vi "AnalogIntegrator_NI5771.vi"() -> ()   [LabVIEW 2012]
uses:
  <vilib>/Platform/TimedLoop/XDataNode/timing_clust.ctl
  <vilib>/Platform/TimedLoop/XDataNode/nitl_modes.ctl
  <vilib>/Platform/TimedLoop/XDataNode/wakeup.ctl
  <vilib>/rvi/FIFO/Fifo_Resource/nirvififoEmulationSetSize.vi
  <vilib>/rvi/DataTransferAndStorage/Container/Common/niFpgaContainerGetUniqueNameForEmu.vi
  <vilib>/rvi/eio/common/nirviEmuTemplateMethod_errors.vi
  <vilib>/rvi/Emulation/niFpgaSctlEmulationRegisterWithScheduler.vi
  <vilib>/rvi/errors/niFpgaSetErrorForExecOnDevCompSimple.vi
  <vilib>/rvi/eio/common/nirviEmuReportErrorAndStop.vi
  <vilib>/rvi/Emulation/niFpgaSctlEmulationFifoFullMgr.vi
  <vilib>/rvi/Emulation/niFpgaSctlEmulationResourceMgr.vi
  <vilib>/rvi/Emulation/niFpgaSctlEmulationScheduler.vi
  <vilib>/rvi/interface/RandomDataEmulation/nirviRandomDataFPGAFIFO.vi
  <vilib>/rvi/interface/RandomDataEmulation/niFpgaRandomDataHandleErrors.vi
  <vilib>/rvi/Emulation/niFpgaSctlEmulationGlobalWrite.vi
  <vilib>/Platform/TimedLoop/XDataNode/XDataNode.xnode
  <vilib>/rvi/DataTransferAndStorage/Container/XNode/niFpgaContainer.xnode
  <vilib>/rvi/FIFO/Fifo_Resource/nirvififoEmulationClear.vi
  <vilib>/eio/EIONode/EIONode.xnode
  <vilib>/rvi/FIFO/Fifo_Resource/nirvififoEmulationWrite.vi
  <vilib>/rvi/FIFO/Fifo_Resource/nirvififoEmulationRead.vi
  <vilib>/rvi/interface/RandomDataEmulation/nirviRandomDataFpgaReadWriteTemplate.vi
  <vilib>/Platform/TimedLoop/XDataNode/XDNodeRunTimeDep.lvlib
panel:
  in  "Baselinex8 Ch2":u8
  in  "Baselinex8 Ch1":u8
  in  "Clear Interloop FIFO":bool
  out "InterloopFIFO Timeout":bool
  out "ToHostCh2FIFO Overflow":bool
  out "ToHostCh1FIFO Overflow":bool
  out "Pixel counter":u32
  in  "Wait for trigger":bool
  in  "Acquire":bool
  in  "Acquire continuously":bool=TRUE
  in  "Requested pixels":u32=100000
  out "InterloopFIFO Overflow":bool
  out "Acquiring":bool
  out "IO Module\\AI Over Range":bool
  in  "Samples per pixel":u32=10000 caption="Samples per pixel Acq"
  in  "Samples per line":u32=10000 caption="Samples per pixel Acq"
  in  "User Command Commit":bool
  in  "User Command":u8
  out "User Command Idle":bool
  out "User Command Status":u8
  in  "User Data 0":u16
  in  "User Data 1":u8
  out "PLL Locked":bool
  out "User Error":bool
  out "Configured?":bool
  # "5771 IO module configuration"
  # "Analog integrator"
  # "Acquisition control"
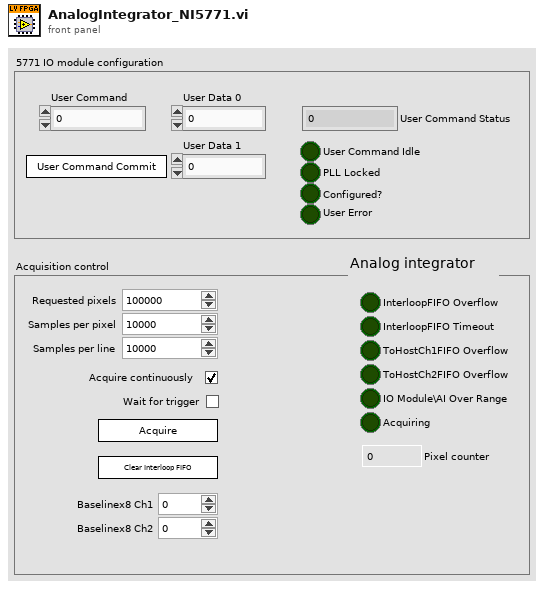
[diagram p1: front panel]
types:
  T1 = typedef "XDNodeRunTimeDep.lvlib/timing_clust.ctl" = cluster{"Expected End [f-1]":u64, "Actual End [f-1]":u64, "Finished Late? [f-1]":bool, "Expected End [i-1]":u64, "Actual End [i-1]":u64, "Finished Late? [i-1]":bool, "Expected Start [i]":u64, "Actual Start [i]":u64, "Expected Start [f]":u64, "Actual Start [f]":u64, "Source Name":string, "Structure Name":string, "Period":i64, "Deadline":i64, "Offset":i64, "Start":i64, "Priority":i32, "Timeout":i32, "Mode":T2, "Wakeup Reason":T3, "Error":errorcluster, "Source Type":string, "Secondary Source Type":string, "Global End Time":u64, "Global Start Time":u64, "Frame Duration":u64, "Iteration Duration":u64, "Assigned CPU":i32, "I/O Scan Engine Mode":u32}
  T2 = typedef "XDNodeRunTimeDep.lvlib/nitl_modes.ctl" = enum32{"No Change", "Process missed periods, maintain original phase", "Discard missed periods, maintain original phase", "Process missed periods, ignore original phase", "Discard missed periods, ignore original phase"}
  T3 = typedef "XDNodeRunTimeDep.lvlib/wakeup.ctl" = enum32{"Normal", "Aborted", "Asynchronous wakeup", "Timing source error", "Timed loop error", "Timeout"}
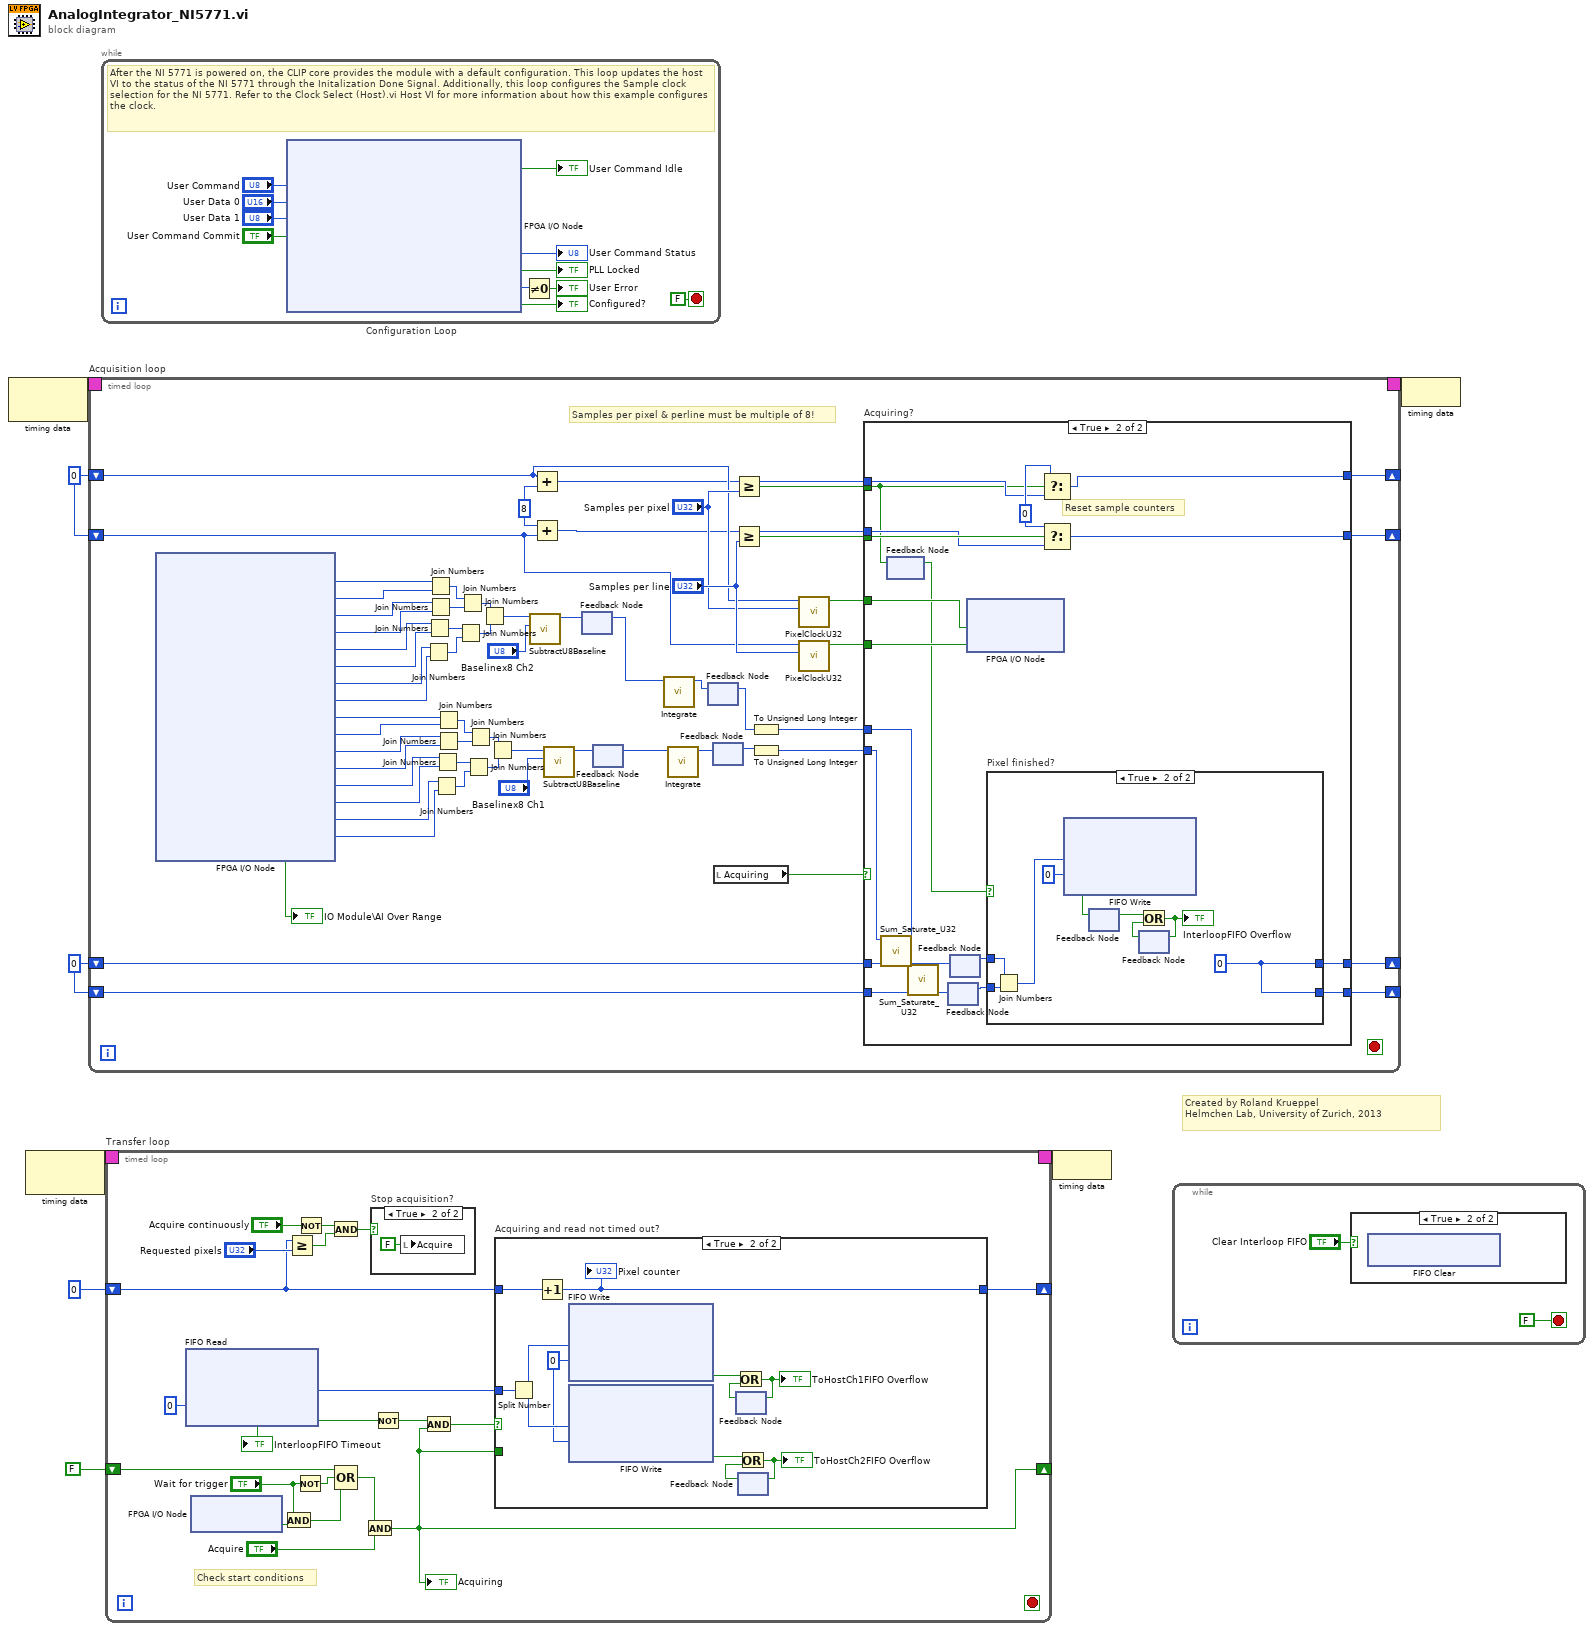
[diagram p0: block diagram]
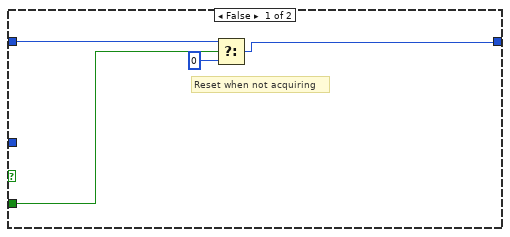
[diagram p4: hidden frame]
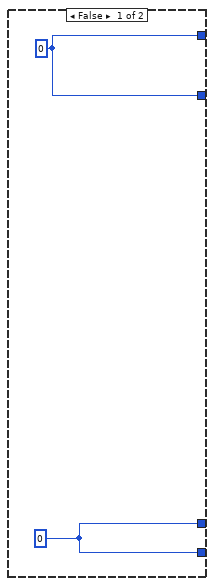
[diagram p5: hidden frame]
diagram:
  w5 = u32 0
  w6 = u32 0 ("t")
  # "Created by Roland Krueppel\nHelmchen Lab, University of Zurich, 2013"
  n1 = node-c288() -> (w8:T1)  [unwired: 1 in]
  n2 = node-c288() -> (w4:T1)  [unwired: 1 in]
  n3 = timed-loop "Acquisition loop" {
    timing: w8 -> [_]
    timing-out: [_] -> w7
    shift-right: [w68] -> _
    shift-left: w6 -> [w57]
    shift-right: [w69] -> _
    shift-left: w6 -> [w56]
    shift-right: [w64] -> _
    shift-left: w5 -> [w66]
    shift-right: [w63] -> _
    shift-left: w5 -> [w65]
    stop <- _ stop-if-true
    w60 = u32 8 ("y")
    # "Samples per pixel & perline must be multiple of 8!"
    n4 = xnode "FPGA I/O Node"() -> ("IO Module\\AI 1 Data N-7"=w42:u8, "IO Module\\AI 1 Data N-6"=w41:u8, "IO Module\\AI 1 Data N-5"=w40:u8, "IO Module\\AI 1 Data N-4"=w39:u8, "IO Module\\AI 1 Data N-3"=w38:u8, "IO Module\\AI 1 Data N-2"=w37:u8, "IO Module\\AI 1 Data N-1"=w36:u8, "IO Module\\AI 1 Data N"=w35:u8, "IO Module\\AI 0 Data N-7"=w28:u8, "IO Module\\AI 0 Data N-6"=w27:u8, "IO Module\\AI 0 Data N-5"=w26:u8, "IO Module\\AI 0 Data N-4"=w25:u8, "IO Module\\AI 0 Data N-3"=w24:u8, "IO Module\\AI 0 Data N-2"=w23:u8, "IO Module\\AI 0 Data N-1"=w22:u8, "IO Module\\AI 0 Data N"=w21:u8, "IO Module\\AI Over Range"=→"IO Module\\AI Over Range":bool)  [unwired: 17 in, 17 out]
    n5 = Join Numbers(hi=w36, lo=w35) -> ((hi.lo)=w46:u16)
    n6 = Join Numbers(hi=w38, lo=w37) -> ((hi.lo)=w45:u16)
    n7 = Join Numbers(hi=w42, lo=w41) -> ((hi.lo)=w43:u16)
    n8 = Join Numbers(hi=w40, lo=w39) -> ((hi.lo)=w44:u16)
    n9 = Join Numbers(hi=w22, lo=w21) -> ((hi.lo)=w32:u16)
    n10 = Join Numbers(hi=w24, lo=w23) -> ((hi.lo)=w31:u16)
    n11 = Join Numbers(hi=w28, lo=w27) -> ((hi.lo)=w29:u16)
    n12 = Join Numbers(hi=w26, lo=w25) -> ((hi.lo)=w30:u16)
    n13 = Join Numbers(hi=w45, lo=w46) -> ((hi.lo)=w48:u32)
    n14 = Join Numbers(hi=w43, lo=w44) -> ((hi.lo)=w47:u32)
    n15 = Join Numbers(hi=w31, lo=w32) -> ((hi.lo)=w34:u32)
    n16 = Join Numbers(hi=w29, lo=w30) -> ((hi.lo)=w33:u32)
    n17 = Join Numbers(hi=w47, lo=w48) -> ((hi.lo)=w19:u64)
    n18 = Join Numbers(hi=w33, lo=w34) -> ((hi.lo)=w18:u64)
    n19 = call "SubtractU8Baseline.vi"("Baseline U8"="Baselinex8 Ch2", "New samples in"=w19) -> ("New samples out"=w13:u64)  [unwired: 9 in]
    n20 = Add(x=w56, y=w60) -> (x+y=w53:u32)
    n21 = Add(x=w60, y=w57) -> (x+y=w51:u32)
    n22 = call "SubtractU8Baseline.vi"("Baseline U8"="Baselinex8 Ch1", "New samples in"=w18) -> ("New samples out"=w16:u64)  [unwired: 9 in]
    n23 = feedback-in #1(w13) -> ()
    n24 = feedback #1() -> (w14:u64)  [unwired: 1 in]
    n25 = feedback #2() -> (w15:u64)  [unwired: 1 in]
    n26 = feedback-in #2(w16) -> ()
    n27 = call "Integrate.vi"("New samples in"=w14) -> ("Sum out"=w12:u16)  [unwired: 9 in, 1 out]
    n28 = call "Integrate.vi"("New samples in"=w15) -> ("Sum out"=w10:u16)  [unwired: 9 in, 1 out]
    n29 = feedback #3() -> (w11:u16)  [unwired: 1 in]
    n30 = feedback-in #3(w12) -> ()
    n31 = feedback #4() -> (w9:u16)  [unwired: 1 in]
    n32 = feedback-in #4(w10) -> ()
    n33 = local read "Acquiring"() -> (w67:bool)
    n34 = Greater Or Equal?(x=w53, y="Samples per pixel") -> (x >= y?=w52:bool)
    n35 = Greater Or Equal?(x=w51, y="Samples per line") -> (x >= y?=w50:bool)
    n36 = To Unsigned Long Integer(number=w11) -> (unsigned 32bit integer=w55:u32)
    n37 = To Unsigned Long Integer(number=w9) -> (unsigned 32bit integer=w54:u32)
    n38 = call "PixelClockU32.vi"("Samples per pixel"="Samples per pixel", "Sample counter"=w56) -> ("Pixel clock"=w59:bool)  [unwired: 9 in]
    n39 = call "PixelClockU32.vi"("Samples per pixel"="Samples per line", "Sample counter"=w57) -> ("Pixel clock"=w58:bool)  [unwired: 9 in]
    n40 = case "Acquiring?" shown="True" w67 {
      tunnel: [w71 w90] -> w69
      tunnel: [w71 w89] -> w68
      tunnel: w54 -> [_ w76]
      tunnel: w66 -> [_ w79]
      tunnel: w65 -> [_ w75]
      tunnel: w55 -> [_ w74]
      tunnel: [w70 w88] -> w64
      tunnel: [w70 w87] -> w63
      tunnel: w52 -> [_ w81]
      tunnel: w50 -> [_ w86]
      tunnel: w53 -> [_ w85]
      tunnel: w51 -> [_ w84]
      tunnel: w59 -> [_ w83]
      tunnel: w58 -> [_ w82]
      frame False {
        w70 = u32 0
        w71 = u16 0 ("t")
      }
      frame True {
        w91 = u32 0 ("t")
        # "Reset sample counters"
        n41 = call "Sum_Saturate_U32.vi"("Sum In"=w79, "New Value"=w76) -> ("Sum Out"=w78:u32)  [unwired: 9 in]
        n42 = feedback #5() -> (w80:bool)  [unwired: 1 in]
        n43 = feedback-in #5(w81) -> ()
        n44 = call "Sum_Saturate_U32.vi"("Sum In"=w75, "New Value"=w74) -> ("Sum Out"=w73:u32)  [unwired: 9 in]
        n45 = feedback #6() -> (w72:u32)  [unwired: 1 in]
        n46 = feedback-in #6(w73) -> ()
        n47 = feedback #7() -> (w77:u32)  [unwired: 1 in]
        n48 = feedback-in #7(w78) -> ()
        n49 = xnode "FPGA I/O Node"("PixelClock"=w83, "LineClock"=w82) -> ()  [unwired: 2 in, 2 out]
        n50 = case "Pixel finished?" shown="True" w80 {
          tunnel: w72 -> [w92 w102]
          tunnel: w77 -> [w93 w101]
          tunnel: [w93 w96] -> w88
          tunnel: [w92 w96] -> w87
          frame False {
          }
          frame True {
            w96 = u32 0
            n51 = Join Numbers(hi=w101, lo=w102) -> ((hi.lo)=w100:u64)
            n52 = xnode ("FIFO Write")("Element"=w100, "Timeout"=0) -> ("Timed Out?"=w94:bool)  [unwired: 1 in, 1 out]
            n53 = feedback-in #8(w94) -> ()
            n54 = feedback #8() -> (w95:bool)  [unwired: 1 in]
            n55 = feedback #9() -> (w97:bool)  [unwired: 1 in]
            n56 = Or(x=w95, y=w97) -> (x .or. y?=w98:bool)
            "InterloopFIFO Overflow" <- w98
            n57 = feedback-in #9(w98) -> ()
          }
        }
        n58 = Select(t=w91, s=w81, f=w85) -> (s? t:f=w90:u32)
        n59 = Select(t=w91, s=w86, f=w84) -> (s? t:f=w89:u32)
      }
    }
  }
  n60 = while "Configuration Loop" {
    stop <- FALSE stop-if-true
    # "After the NI 5771 is powered on, the CLIP core provides the module with a default configuration. This loop updates the host VI to the status of the NI 5771 through the Initalization Done Signal. Additionally, this loop configures the Sample clock selection for the NI 5771. Refer to the Clock Select (Host).vi Host VI for more information about how this example configures the clock."
    n61 = xnode "FPGA I/O Node"("IO Module\\User Command"="User Command", "IO Module\\User Data 0"="User Data 0", "IO Module\\User Data 1"="User Data 1", "IO Module\\User Command Commit"="User Command Commit") -> ("IO Module\\User Command Idle"=→"User Command Idle":bool, "IO Module\\User Command Status"=→"User Command Status":u8, "IO Module\\PLL Locked"=→"PLL Locked":bool, "IO Module\\User Error"=w108:u8, "IO Module\\Initialization Done"=→"Configured?":bool)  [unwired: 9 in, 9 out]
    n62 = Not Equal To 0?(x=w108) -> (x != 0?=→"User Error":bool)
  }
  n63 = timed-loop "Transfer loop" {
    timing: w4 -> [_]
    timing-out: [_] -> w3
    shift-right: [w118] -> _
    shift-left: u32 0 -> [w119]
    shift-right: [w117] -> _
    shift-left: FALSE -> [w125]
    stop <- _ stop-if-true
    # "Check start conditions"
    n64 = xnode ("FIFO Read")("Timeout"=0) -> ("Element"=w120:u64, "Timed Out?"=w124:bool)  [unwired: 1 in, 1 out]
    "InterloopFIFO Timeout" <- w124
    n65 = xnode "FPGA I/O Node"() -> ("TriggerIn"=w130:bool)  [unwired: 1 in, 1 out]
    n66 = And(x="Wait for trigger", y=w130) -> (x .and. y?=w127:bool)
    n67 = Greater Or Equal?(x=w119, y="Requested pixels") -> (x >= y?=w132:bool)
    n68 = Not(x="Wait for trigger") -> (.not. x?=w128:bool)
    n69 = Not(x="Acquire continuously") -> (.not. x?=w133:bool)
    n70 = And(x=w133, y=w132) -> (x .and. y?=w122:bool)
    n71 = Compound Arithmetic op=OR(w125, w128, w127) -> (w126:bool)
    n72 = And(x=w126, y="Acquire") -> (x .and. y?=w117:bool)
    "Acquiring" <- w117
    n73 = case "Stop acquisition?" shown="True" w122 {
      frame False {
      }
      frame True {
        n74 = local write "Acquire"(FALSE ("Acquire")) -> ()
      }
    }
    n75 = Not(x=w124) -> (.not. x?=w123:bool)
    n76 = And(x=w123, y=w117) -> (x .and. y?=w121:bool)
    n77 = case "Acquiring and read not timed out?" shown="True" w121 {
      tunnel: w120 -> [_ w152]
      tunnel: w119 -> [w139 w148]
      tunnel: [w138 w147] -> w118
      tunnel: w117 -> [w140 _]
      frame False {
        # "Reset when not acquiring"
        n78 = Select(t=w139, s=w140, f=u32 0) -> (s? t:f=w138:u32)
      }
      frame True {
        w149 = 0 ("Timeout")
        n79 = Split Number(x=w152) -> (hi(x)=w151:u32, lo(x)=w150:u32)
        n80 = Increment(x=w148) -> (x+1=w147:u32)
        "Pixel counter" <- w147
        n81 = xnode ("FIFO Write")("Element"=w151, "Timeout"=w149) -> ("Timed Out?"=w145:bool)  [unwired: 1 in, 1 out]
        n82 = xnode ("FIFO Write")("Element"=w150, "Timeout"=w149) -> ("Timed Out?"=w142:bool)  [unwired: 1 in, 1 out]
        n83 = feedback #10() -> (w144:bool)  [unwired: 1 in]
        n84 = Or(x=w145, y=w144) -> (x .or. y?=w146:bool)
        "ToHostCh1FIFO Overflow" <- w146
        n85 = feedback-in #10(w146) -> ()
        n86 = feedback #11() -> (w141:bool)  [unwired: 1 in]
        n87 = Or(x=w142, y=w141) -> (x .or. y?=w143:bool)
        "ToHostCh2FIFO Overflow" <- w143
        n88 = feedback-in #11(w143) -> ()
      }
    }
  }
  n89 = node-c288(w3) -> ()
  n90 = while {
    stop <- FALSE stop-if-true
    n91 = case shown="True" "Clear Interloop FIFO" {
      frame False {
      }
      frame True {
        n92 = xnode ("FIFO Clear")() -> ()  [unwired: 1 in, 1 out]
      }
    }
  }
  n93 = node-c288(w7) -> ()
